vi "Get FK Columns.vi"(8 "error in (no error)":errorcluster, 11 "Table Configuration in":refnum<class "Table Configuration.lvclass">) -> (0 "error out":errorcluster, 2 "FKs":map{string, T1}(c390), 3 "Table Configuration out":refnum<class "Table Configuration.lvclass">)   [LabVIEW 2020, in "Table.lvlib" / "Table Configuration.lvclass"]
uses:
  Table Configuration.lvclass
  Column Libraries/Column Interface/FK Info.ctl
  Table Configuration.lvclass/Table Configuration.ctl
  Column Libraries/Column Interfaces.lvlib
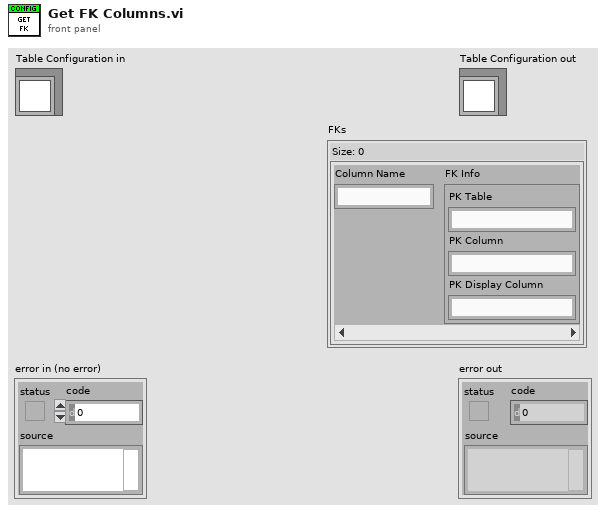
[diagram p1: front panel]
types:
  T1 = typedef "Column Interfaces.lvlib/FK Info.ctl" = cluster{"PK Table":string, "PK Column":string, "PK Display Column":string}
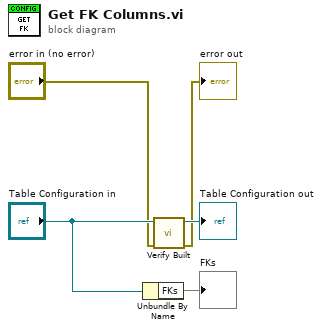
[diagram p0: block diagram]
diagram:
  n1 = Unbundle By Name("Table Configuration in") -> ("FKs"=→"FKs":map{string, T1})
  n2 = call-dynamic "Verify Built.vi"("error in (no error)"="error in (no error)", "Table Configuration in"="Table Configuration in") -> ("error out"=→"error out":errorcluster, "Table Configuration out"=→"Table Configuration out":refnum<class "Table Configuration.lvclass">)  [unwired: 8 in]
